vi "get chassis information.vi"(6 "detect modules (T)":bool=TRUE, 8 "error in":errorcluster, 11 "controller in":refnum<class "Controller.lvclass">) -> (0 "error out":errorcluster, 1 "remote chassis":T1[](array[typedef]) {"chassis"."product ID" format="%.0x"; "modules"."product ID" format="%.0x"}, 2 "local chassis":T1[](array[typedef]) {"chassis"."product ID" format="%.0x"; "modules"."product ID" format="%.0x"}, 3 "controller out":refnum<class "Controller.lvclass">)   [LabVIEW 2014, in "SMI.lvlib" / "Chassis.lvclass"]
uses:
  Chassis.lvclass
  Controller/Controller.lvclass
  chassis and module information.ctl
  chassis information.ctl
  Module/module information.ctl
  Chassis.lvclass/Chassis.ctl
  Device/read device class.vi
  Device/read serial number.vi
  Device/read product ID.vi
  Device/read product name.vi
  Device/read vendor name.vi
  Controller/read remote chassis.vi
  Controller/read local chassis.vi
  Module/Module.lvclass
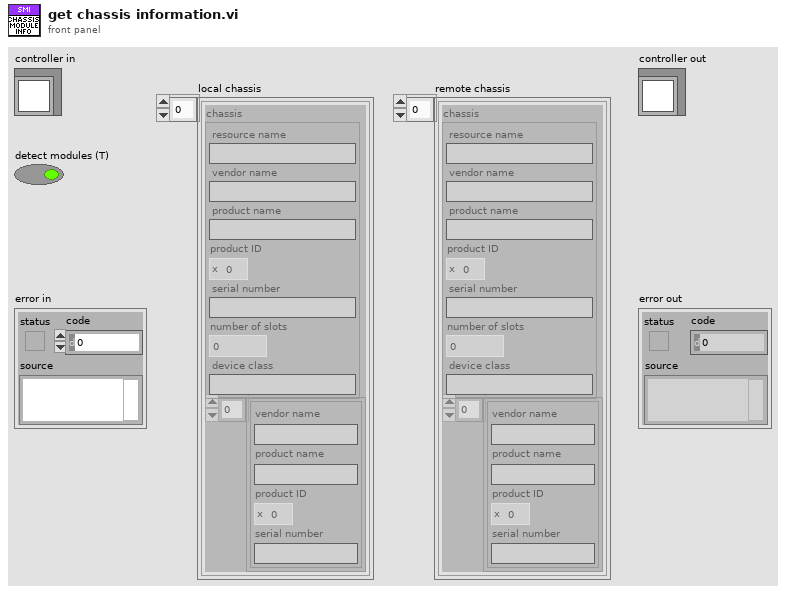
[diagram p1: front panel]
types:
  T1 = typedef "SMI.lvlib/Chassis.lvclass/chassis and module information.ctl" = cluster{"chassis":T2, "modules":T3[]}
  T2 = typedef "SMI.lvlib/Chassis.lvclass/chassis information.ctl" = cluster{"resource name":string, "vendor name":string, "product name":string, "product ID":u16, "serial number":string, "number of slots":i32, "device class":string}
  T3 = typedef "SMI.lvlib/Module.lvclass/module information.ctl" = cluster{"vendor name":string, "product name":string, "product ID":u16, "serial number":string}
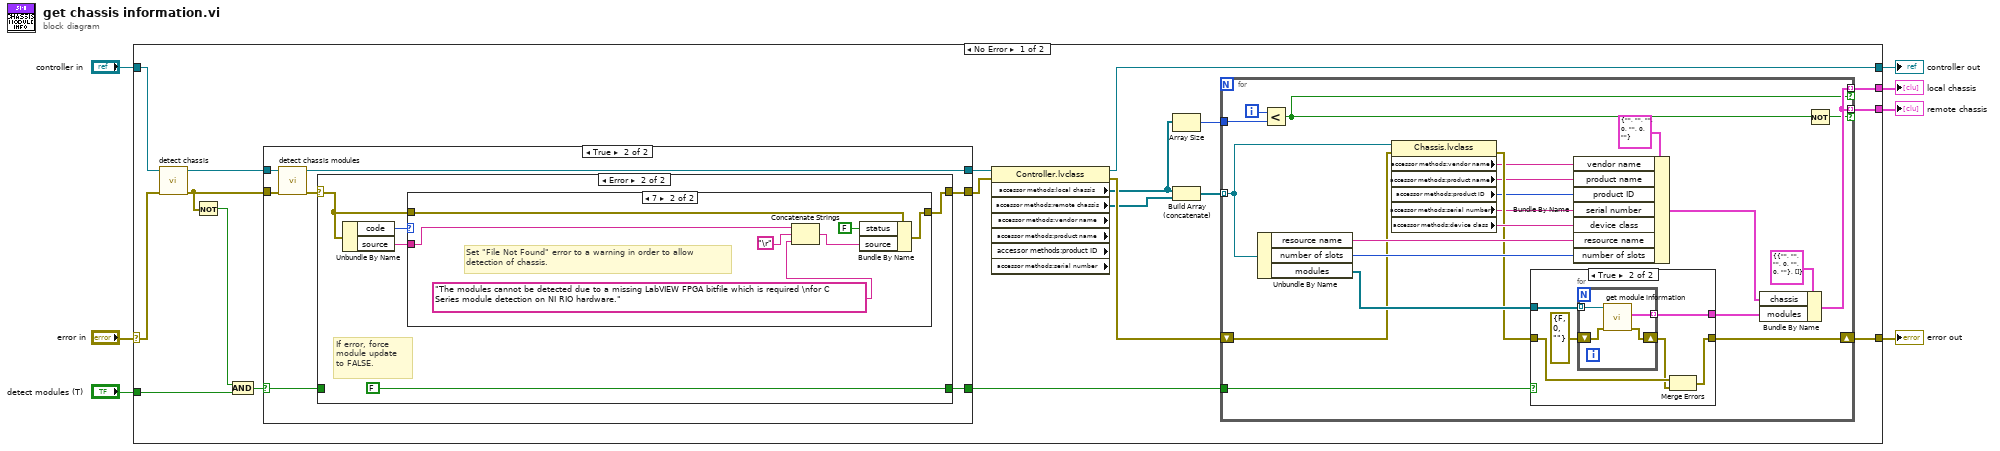
[diagram p0: block diagram]
diagram:
  n1 = case shown="No Error" "error in" {
    selector: "error in" -> [w10 w85]
    tunnel: [w25 w86] -> w7
    tunnel: [w20 w85] -> w6
    tunnel: "controller in" -> [w9 w86]
    tunnel: [w16 _] -> w5
    tunnel: [w15 _] -> w4
    tunnel: "detect modules (T)" -> [w11 _]
    frame No Error {
      n2 = call "detect chassis.vi"("error in"=w10, "controller in"=w9) -> ("error out"=w13:errorcluster, "controller out"=w12:refnum<class "Controller.lvclass">)  [unwired: 8 in]
      n3 = Not(x=w13) -> (.not. x?=w8:bool)
      n4 = And(x=w8, y=w11) -> (x .and. y?=w14:bool)
      n5 = case shown="True" w14 {
        selector: w14 -> [w27 w30]
        tunnel: w13 -> [w28 w36]
        tunnel: w12 -> [w29 w35]
        tunnel: [w29 w34] -> w18
        tunnel: [w28 w32] -> w19
        tunnel: [w27 w31] -> w17
        frame False {
        }
        frame True {
          n6 = call "detect chassis modules.vi"("error in"=w36, "controller in"=w35) -> ("error out"=w33:errorcluster, "controller out"=w34:refnum<class "Controller.lvclass">)  [unwired: 8 in]
          n7 = case shown="Error" w33 {
            selector: w33 -> [w38 w42]
            tunnel: [w38 w40] -> w32
            tunnel: w30 -> [w37 _]
            tunnel: [w37 FALSE ("detect modules (T)")] -> w31
            frame No Error {
            }
            frame Error {
              # "If error, force \nmodule update \nto FALSE."
              n8 = Unbundle By Name(w42) -> ("code"=w43:i32, "source"=w41:string)
              n9 = case shown="7" w43 {
                tunnel: w42 -> [w44 w51]
                tunnel: w41 -> [_ w49]
                tunnel: [w44 w45] -> w40
                frame Default {
                }
                frame 7 {
                  # "Set \"File Not Found\" error to a warning in order to allow\ndetection of chassis."
                  n10 = Concatenate Strings(w49, "\r", "The modules cannot be detected due to a missing LabVIEW FPGA bitfile which is required \nfor C Series module detection on NI RIO hardware." ("message")) -> (w46:string)
                  n11 = Bundle By Name(cluster=w51, "status"=FALSE, "source"=w46) -> (w45:errorcluster)
                }
              }
            }
          }
        }
      }
      n12 = property class="Controller.lvclass" props=["accessor methods:local chassis", "accessor methods:remote chassis", "accessor methods:vendor name", "accessor methods:product name", "accessor methods:product ID", "accessor methods:serial number"](reference=w18, error in=w19) -> (reference out=w25:refnum<class "Controller.lvclass">, error out=w26:errorcluster, "accessor methods:local chassis"=w24:refnum<class "Chassis.lvclass">[], "accessor methods:remote chassis"=w23:refnum<class "Chassis.lvclass">[])  [unwired: 4 out]
      n13 = Array Size(array=w24) -> (size(s)=w21:i32)
      n14 = Build Array (concatenate)(w24, w23) -> (w22:refnum<class "Chassis.lvclass">[])
      n15 = for {
        tunnel: w22 -> [w59] mode=indexing
        tunnel: w21 -> [w72]
        tunnel: w17 -> [w70]
        shift-right: [w71] -> w20
        shift-left: w26 -> [w57]
        tunnel: [w69] -> w16 mode=indexing if=w68
        tunnel: [w69] -> w15 mode=indexing if=w67
        i -> [w73]
        n16 = Unbundle By Name(w59) -> ("resource name"=w64:string, "number of slots"=w63:i32, "modules"=w66:refnum<class "Module.lvclass">[])
        n17 = Less?(x=w73, y=w72) -> (x < y?=w68:bool)
        n18 = property class="Chassis.lvclass"(reference=w59, error in=w57) -> (error out=w56:errorcluster, "accessor methods:vendor name"=w52:string, "accessor methods:product name"=w53:string, "accessor methods:product ID"=w54:u16, "accessor methods:serial number"=w55:string, "accessor methods:device class"=w58:string)  [unwired: 1 out]
        n19 = case shown="True" w70 {
          tunnel: w66 -> [_ w80]
          tunnel: [_ w79] -> w60
          tunnel: [w74 w75] -> w71
          tunnel: w56 -> [w74 w77]
          frame False {
          }
          frame True {
            n20 = for {
              tunnel: w80 -> [w84] mode=indexing
              tunnel: [w83] -> w79 mode=indexing
              shift-right: [w81] -> w76
              shift-left: errorcluster {"status"=FALSE, "code"=0, "source"=""} ("error out") -> [w82]
              n21 = call "get module information.vi"("error in"=w82, "Module in"=w84) -> ("error out"=w81:errorcluster, "Module Information"=w83:T3)  [unwired: 7 in, 1 out]
            }
            n22 = Merge Errors(w77, w76) -> (w75:errorcluster)
          }
        }
        n23 = Bundle By Name(cluster=T2 {"resource name"="", "vendor name"="", "product name"="", "product ID"=0, "serial number"="", "number of slots"=0, "device class"=""} ("Chassis Information"), "vendor name"=w52, "product name"=w53, "product ID"=w54, "serial number"=w55, "device class"=w58, "resource name"=w64, "number of slots"=w63) -> (w62:T2)
        n24 = Bundle By Name(cluster=T1 {"chassis"={"resource name"="", "vendor name"="", "product name"="", "product ID"=0, "serial number"="", "number of slots"=0, "device class"=""}, "modules"=[]} ("Chassis Information"), "chassis"=w62, "modules"=w60) -> (w69:T1)
        n25 = Not(x=w68) -> (.not. x?=w67:bool)
      }
    }
    frame Error {
    }
  }
  "error out" <- w6
  "controller out" <- w7
  "local chassis" <- w5
  "remote chassis" <- w4
